vi "niRFUtil MT UTIL Resampling Filter.vi"(0 "interpolation factor in":i32=128, 5 "effective filter length":i32=8, 12 "legacy filter?":bool) -> (4 "filerData[]":T1 min=0 max=127 format="%.2f", 6 "interpolation factor":i32=128, 8 "effective filter length":i32=16)   [LabVIEW 2015, in "niRFUtil.lvlib"]
uses:
  niRFUtil.lvlib
  Includes/niRFUtil INC Real Array.ctl
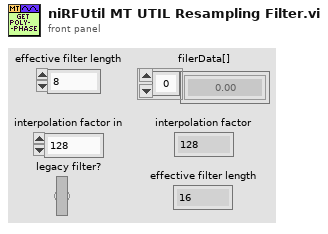
[diagram p1: front panel]
types:
  T1 = typedef "niRFUtil.lvlib/niRFUtil INC Real Array.ctl" = sgl[]
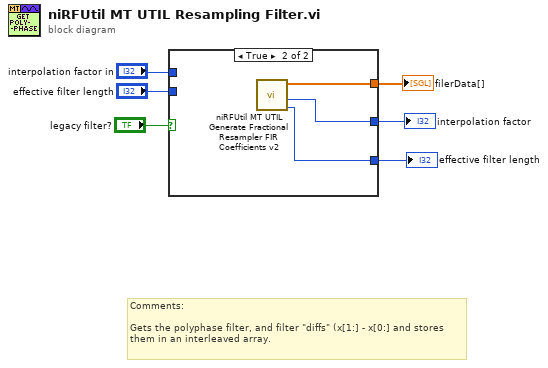
[diagram p0: block diagram]
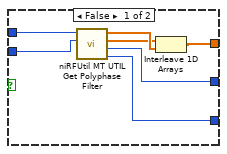
[diagram p2: hidden frame]
diagram:
  # "Comments:\n\nGets the polyphase filter, and filter \"diffs\" (x[1:] - x[0:] and stores\nthem in an interleaved array."
  n1 = case shown="True" "legacy filter?" {
    tunnel: [w11 w16] -> w6
    tunnel: "interpolation factor in" -> [w10 _]
    tunnel: "effective filter length" -> [w9 _]
    tunnel: [w8 w15] -> w3
    tunnel: [w7 w14] -> w2
    frame False {
      n2 = call "niRFUtil MT UTIL Get Polyphase Filter.vi"("# of zero crossings"=w9, "interpolation factor in"=w10) -> ("effective filter length"=w7:i32, "interpolation factor"=w8:i32, "differencesBetweenCoeffs[]"=w12:T1, "scaledFilterCoefficients[]"=w13:T1)  [unwired: 1 in, 5 out]
      n3 = Interleave 1D Arrays(w12, w13) -> (w11:T1)
    }
    frame True {
      n4 = call "niRFUtil MT UTIL Generate Fractional Resampler FIR Coefficients v2.vi"() -> ("effective filter length"=w14:i32, "interpolation factor"=w15:i32, "polyphase filter"=w16:T1)  [unwired: 9 out]
    }
  }
  "filerData[]" <- w6
  "interpolation factor" <- w3
  "effective filter length" <- w2
